vi "Normalize with Highest Den Term (CDB).vi"(10 "Denominator":cdb[](array[numeric]), 11 "Numerator":cdb[](array[numeric])) -> (0 "error":i32, 2 "Normalized Denominator":cdb[](array[numeric]), 3 "Normalized Numerator":cdb[](array[numeric]))   [LabVIEW 2017, in "NI_AALPro.lvlib"]
doc: "Normalizes numerator and denominator polynomials with the highest denominator term. The data types you wire to the <B>Numerator</B> and <B>Denominator</B> inputs determine the polymorphic instance to use."
uses:
  NI_AALPro.lvlib
  Remove Zero Coefficients (CDB).vi
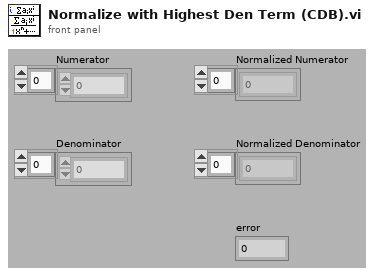
[diagram p1: front panel]
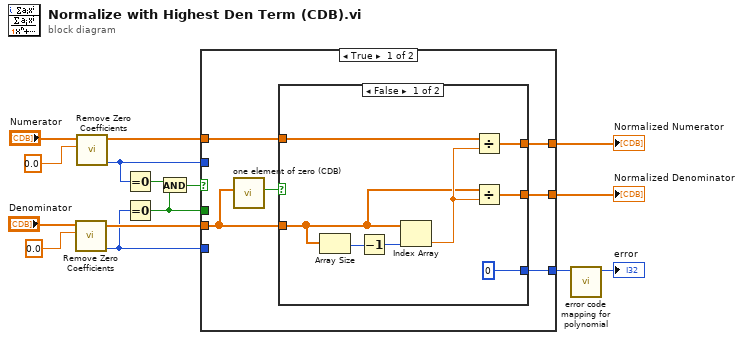
[diagram p0: block diagram]
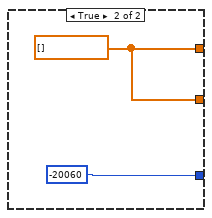
[diagram p2: hidden frame]
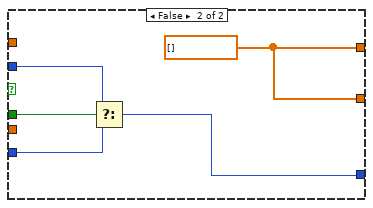
[diagram p3: hidden frame]
diagram:
  n1 = call-poly "Remove Zero Coefficients.vi"("threshold"=0.0, "P(x) In"="Denominator") -> ("error"=w4:i32, "P(x) Out"=w8:cdb[])  [unwired: 7 in, 1 out]
  n2 = call-poly "Remove Zero Coefficients.vi"("threshold"=0.0, "P(x) In"="Numerator") -> ("error"=w5:i32, "P(x) Out"=w11:cdb[])  [unwired: 7 in, 1 out]
  n3 = Equal To 0?(x=w5) -> (x = 0?=w2:bool)
  n4 = Equal To 0?(x=w4) -> (x = 0?=w1:bool)
  n5 = And(x=w2, y=w1) -> (x .and. y?=w3:bool)
  n6 = case shown="True" w3 {
    tunnel: [w21 w36] -> w15
    tunnel: [w20 w36] -> w14
    tunnel: w8 -> [w17 _]
    tunnel: w11 -> [w19 _]
    tunnel: [w18 w33] -> w7
    tunnel: w5 -> [_ w35]
    tunnel: w4 -> [_ w34]
    tunnel: w1 -> [_ w32]
    frame True {
      n7 = call "one element of zero (CDB).vi"("Array in"=w17) -> ("equal [0]?"=w16:bool)  [unwired: 10 in]
      n8 = case shown="False" w16 {
        tunnel: [w29 w31] -> w21
        tunnel: [w28 w31] -> w20
        tunnel: w17 -> [w24 _]
        tunnel: w19 -> [w23 _]
        tunnel: [0 -20060 ("divide by zero")] -> w18
        frame False {
          n9 = Array Size(array=w24) -> (size(s)=w26:i32)
          n10 = Decrement(x=w26) -> (x-1=w25:i32)
          n11 = Index Array(array=w24, index=w25) -> (element=w27:cdb)
          n12 = Divide(x=w23, y=w27) -> (x/y=w28:cdb[])
          n13 = Divide(x=w24, y=w27) -> (x/y=w29:cdb[])
        }
        frame True {
          w31 = cdb[] [] ("BDL")
        }
      }
    }
    frame False {
      w36 = cdb[] [] ("BDL")
      n14 = Select(t=w35, s=w32, f=w34) -> (s? t:f=w33:i32)
    }
  }
  "Normalized Denominator" <- w15
  "Normalized Numerator" <- w14
  n15 = call "error code mapping for polynomial.vi"("error in"=w7) -> ("error out"=→"error":i32)  [unwired: 10 in]
